vi "test_add_ID.vi"() -> ()   [LabVIEW 2023]
uses:
  <vilib>/addons/_JKI Toolkits/Caraya/classes/Assert/Assert Equal Value_Variant.vi
  <vilib>/addons/_JKI Toolkits/Caraya/classes/Assert/Assert Not Error.vi
  <vilib>/addons/_JKI Toolkits/Caraya/classes/Test/Test.lvclass
  <vilib>/addons/_JKI Toolkits/Caraya/classes/Assert/Assert.lvclass
  <vilib>/JDP Science/JSONtext/JSONtext.lvlib
  Source/Classes/Communicator/Communicator.lvclass
panel:
  out "<JSON>":string
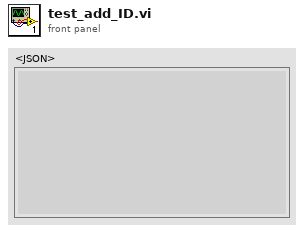
[diagram p1: front panel]
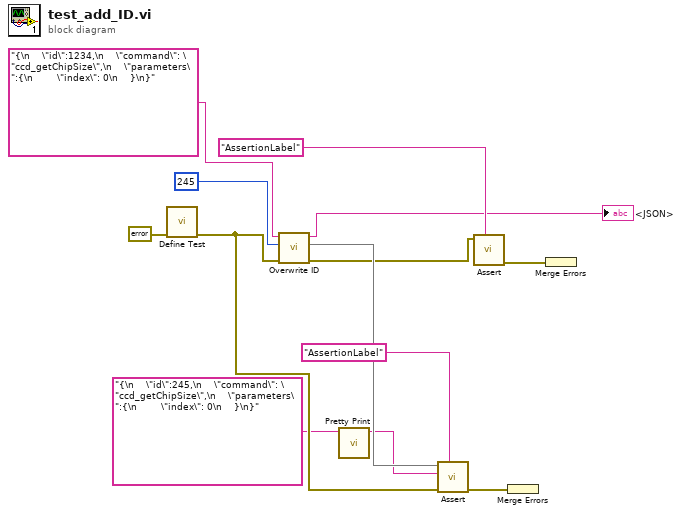
[diagram p0: block diagram]
diagram:
  n1 = call <vilib>:"Define Test.vi"("error in (no error)"=errorcluster {"status"=FALSE, "code"=0, "source"=""}) -> ("error out"=w8:errorcluster)  [unwired: 9 in, 1 out]
  n2 = call "Overwrite ID.vi"("error in (no error)"=w8, "Numeric"=245, "String"="{\n    \"id\":1234,\n    \"command\": \"ccd_getChipSize\",\n    \"parameters\":{\n        \"index\": 0\n    }\n}") -> ("error out"=w1:errorcluster, 2:w4, "<JSON>"=→"<JSON>":string)  [unwired: 6 in]
  n3 = call <vilib>:"Pretty Print.vi"("JSON"="{\n    \"id\":245,\n    \"command\": \"ccd_getChipSize\",\n    \"parameters\":{\n        \"index\": 0\n    }\n}") -> ("<JSON>"=w2:string)  [unwired: 8 in, 2 out]
  n4 = call-poly <vilib>:"Assert.vi"("Label"="AssertionLabel" ("Label (VI Title)"), "error in (no error)"=w8, "Y"=w2, "X"=w4) -> ("error out"=w10:errorcluster)  [unwired: 6 in, 1 out]
  n5 = call-poly <vilib>:"Assert.vi"("Label"="AssertionLabel" ("Label (VI Title)"), "Not Error?"=w1) -> ("error out"=w6:errorcluster)  [unwired: 8 in, 1 out]
  n6 = Merge Errors(w10) -> ()  [unwired: 1 out]
  n7 = Merge Errors(w6) -> ()  [unwired: 1 out]
